vi "Main.vi"() -> ()   [LabVIEW 2020]
doc: "Ce VI modèle est conçu pour le modèle de conception Gestionnaire de messages dans une file d'attente.\n\nLa boucle de gestion d'événements génère des messages en fonction des actions sur l'interface utilisateur.\n\nLa boucle de gestion de messages traite les messages générés par la boucle de gestion d'événements ou par d'autres messages. Les messages sont des valeurs chaîne ; il est donc facile d'ajouter de nouveaux messages à la structure condition Conditions de messages de la boucle de gestion de messages Chaque cluster Message peut en outre fournir une valeur optionnelle pour Données de message, un variant qui peut être converti aux données requises pour un message spécifique."
uses:
  controls/UI Data.ctl
  support/Message Queue/All Message Queues.ctl
  support/Message Queue/Message Cluster.ctl
  controls/Display_Local.ctl
  support/Message Queue/Enqueue Message (Single).vi
  <vilib>/Utility/error.llb/Error Cluster From Error Code.vi
  <vilib>/ErrorRing/Error Ring.xnode
  support/Message Queue/Message Queue.lvlib
  support/User Event - Stop/User Event - Stop.lvlib
panel:
  in  "Cmd_Pad":T1
  in  "BTN_Error":bool
  in  "Btn_Arrêter":bool
  out "Ind_Display":T2
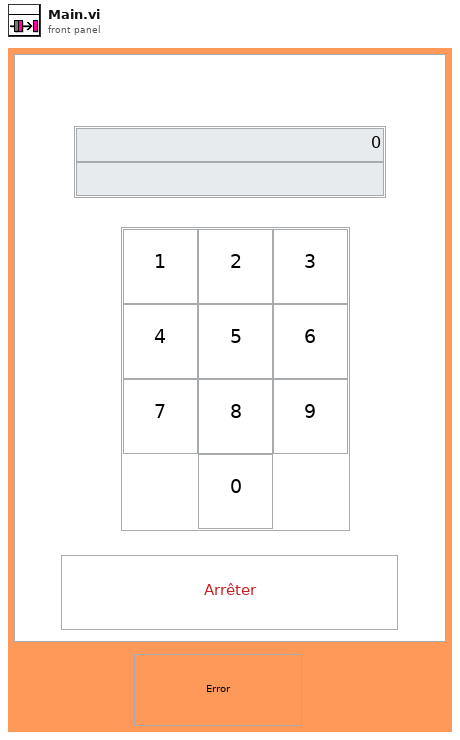
[diagram p1: front panel]
types:
  T1 = cluster{"Btn_1":bool, "Btn_2":bool, "Btn_3":bool, "Btn_4":bool, "Btn_5":bool, "Btn_6":bool, "Btn_7":bool, "Btn_8":bool, "Btn_9":bool, "Btn_10":bool}
  T2 = cluster{"Display_Numérique":dbl, "Display_Chaine":string}
  T3 = cluster{"état":bool, "code":i32, "source":string}
  T4 = typedef "Message Queue.lvlib/All Message Queues.ctl" = cluster{"IU":refnum<queue>, "CO":refnum<queue>}
  T5 = typedef "Display_Local.ctl" = cluster{"Display_Numérique":refnum<vi>, "Display_Chaine":refnum<vi>, "QMH":T4}
  T6 = typedef "UI Data.ctl" = cluster{"Char_Display":string, "Event_Stop ":refnum<user-event>, "QMH":T4}
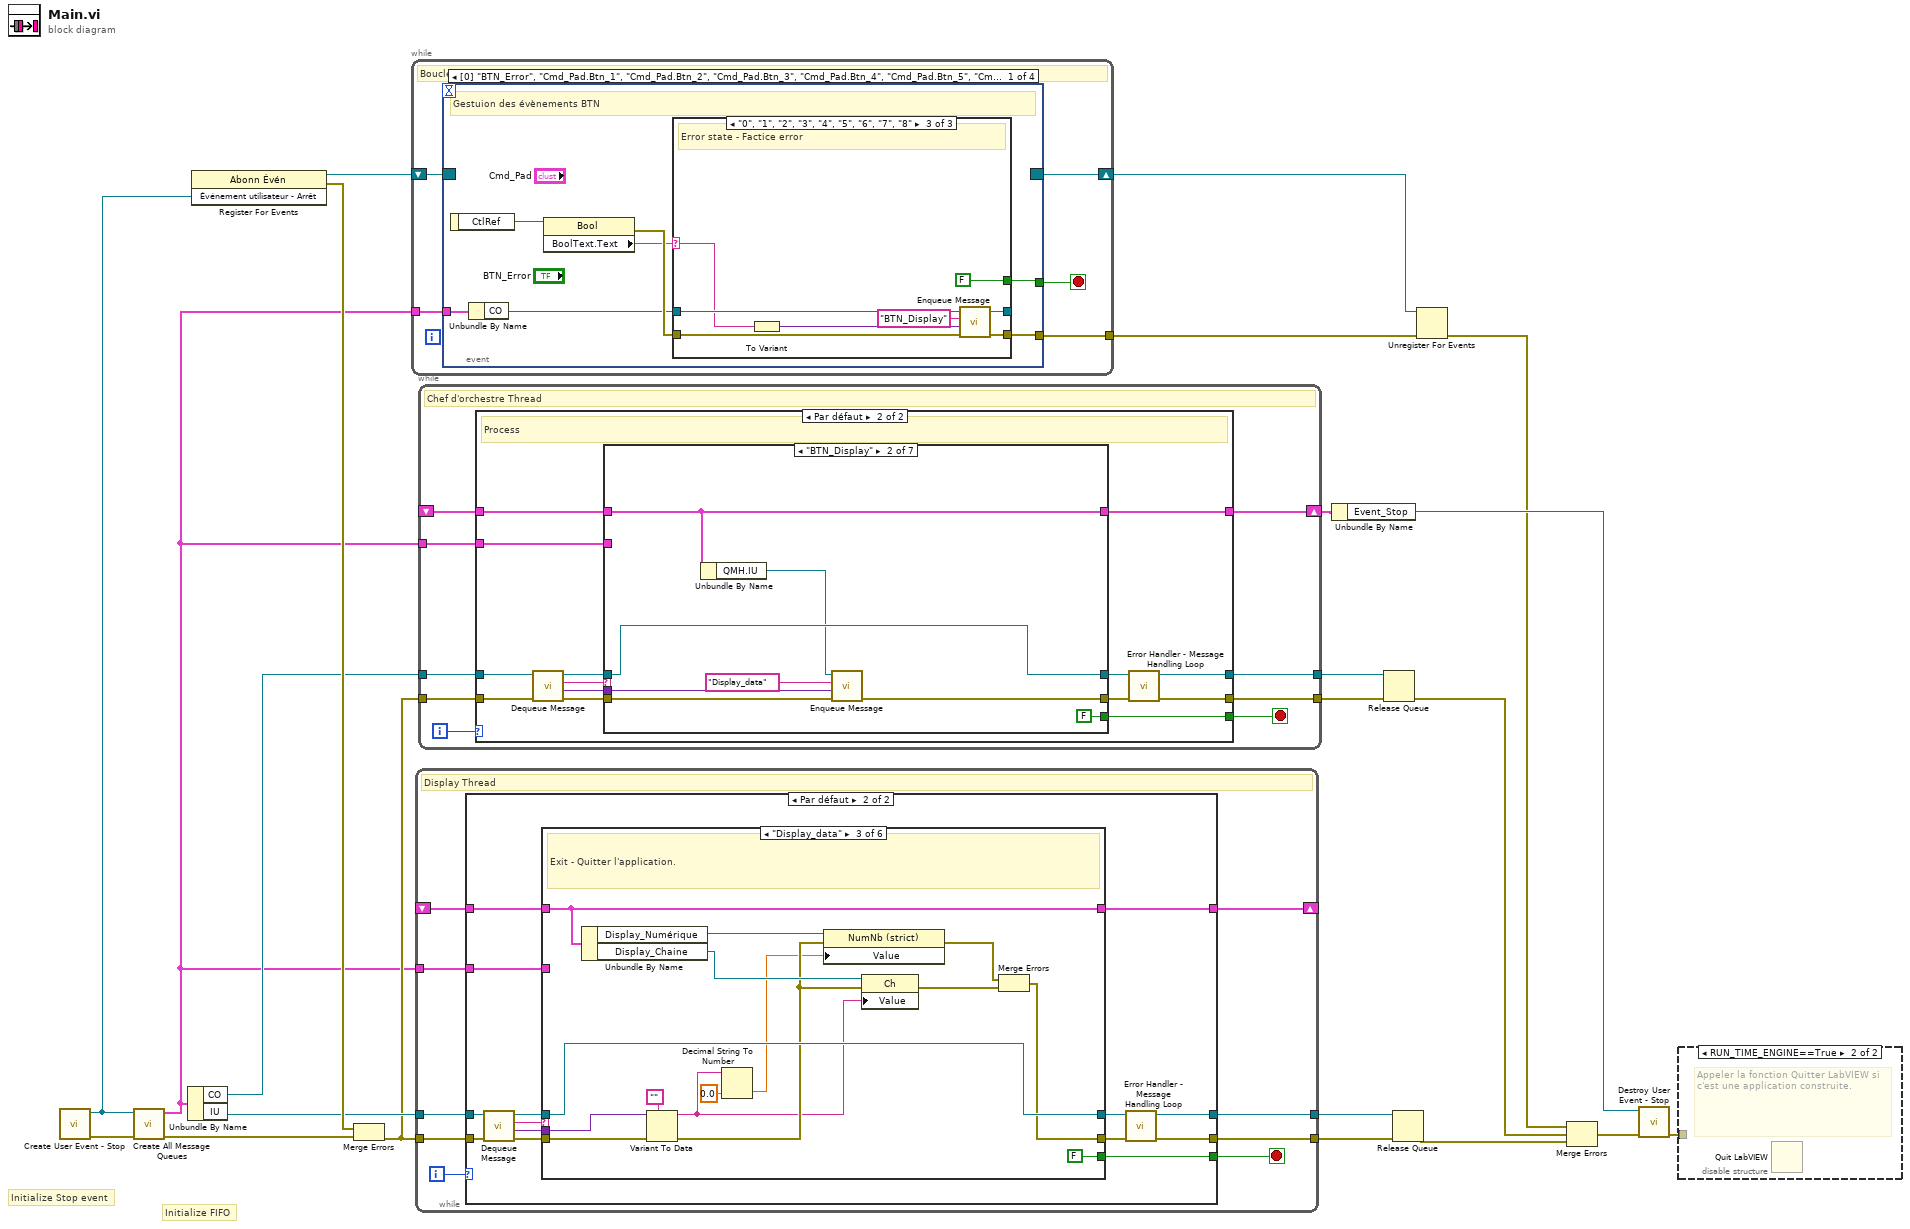
[diagram p0: block diagram]
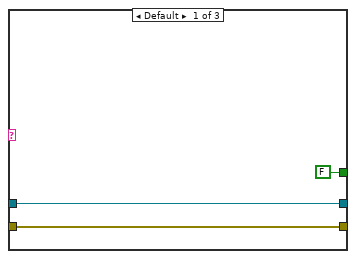
[diagram p2: hidden frame]
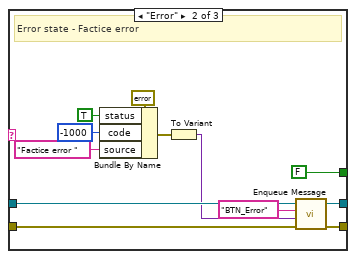
[diagram p3: hidden frame]
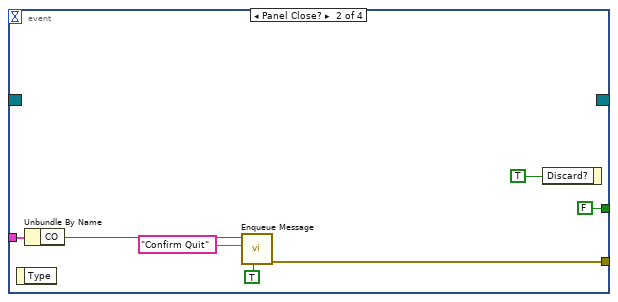
[diagram p4: hidden frame]
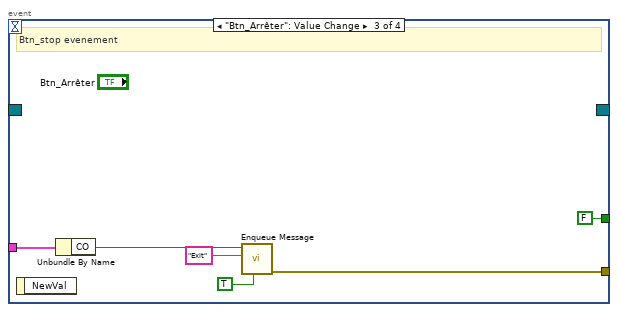
[diagram p5: hidden frame]
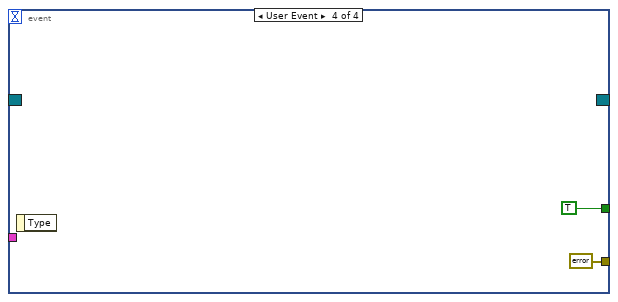
[diagram p6: hidden frame]
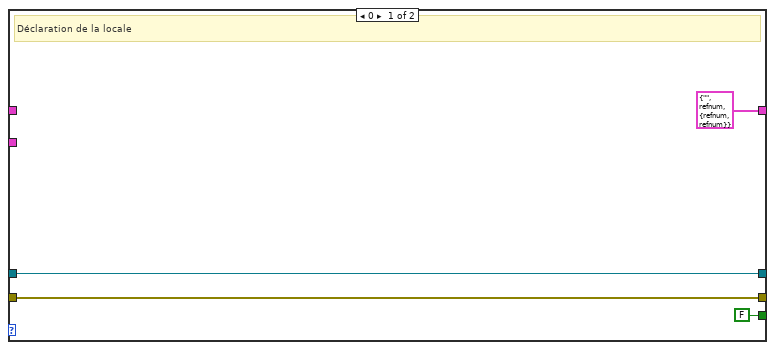
[diagram p7: hidden frame]
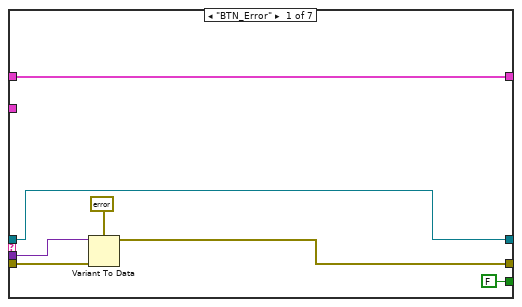
[diagram p8: hidden frame]
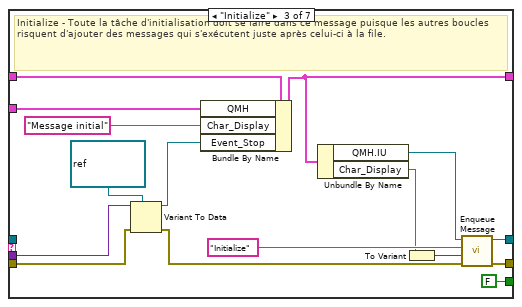
[diagram p9: hidden frame]
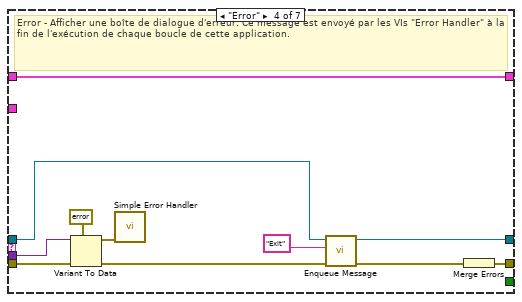
[diagram p10: hidden frame]
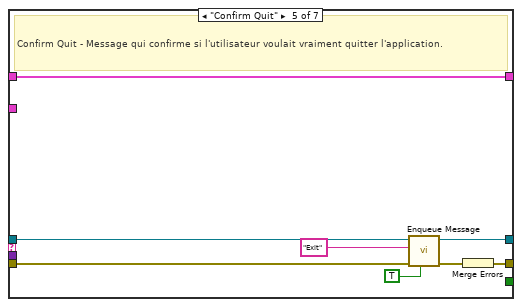
[diagram p11: hidden frame]
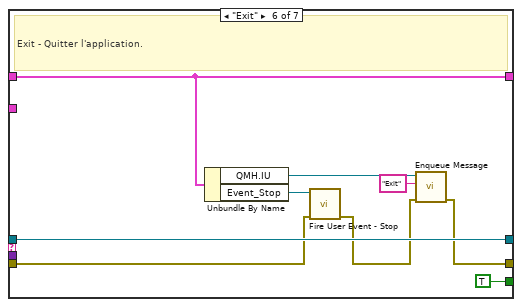
[diagram p12: hidden frame]
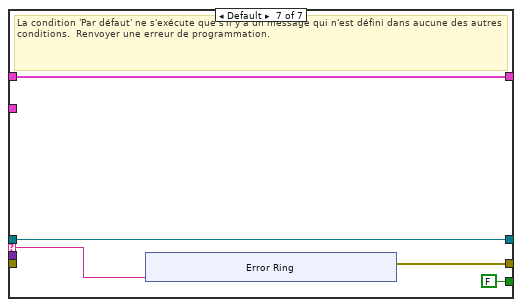
[diagram p13: hidden frame]
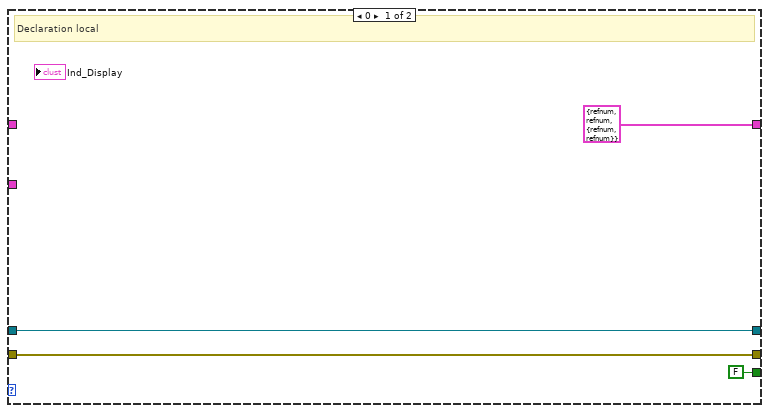
[diagram p14: hidden frame]
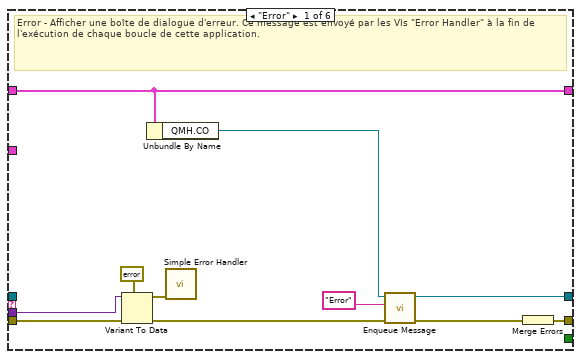
[diagram p15: hidden frame]
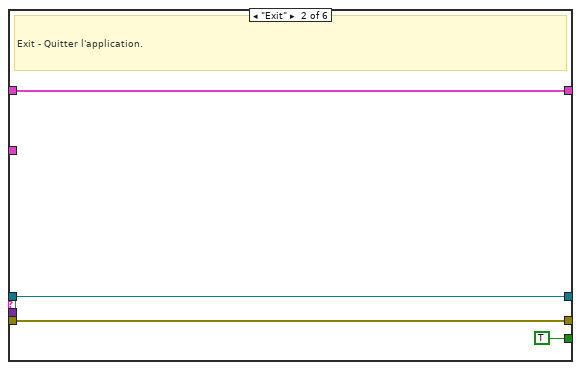
[diagram p16: hidden frame]
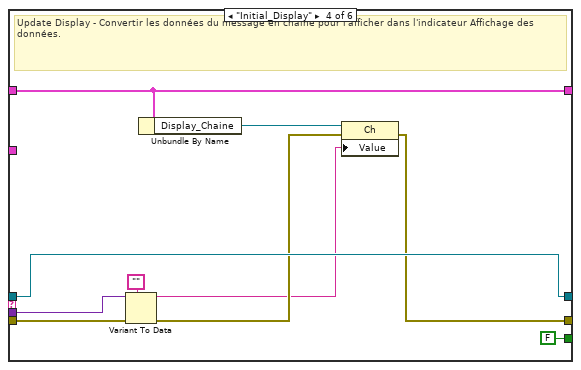
[diagram p17: hidden frame]
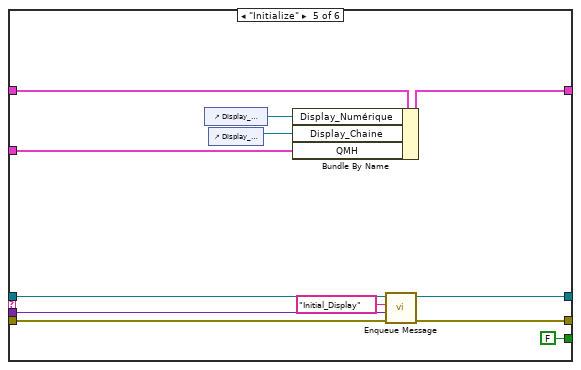
[diagram p18: hidden frame]
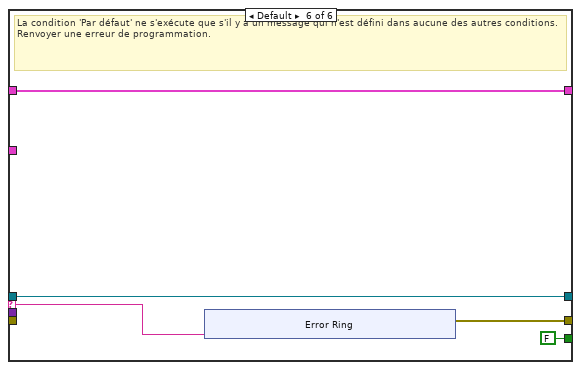
[diagram p19: hidden frame]
diagram:
  # "Initialize FIFO"
  # "Initialize Stop event"
  n1 = call "Create User Event - Stop.vi"() -> ("error out"=w21:T3, "Événement utilisateur - Arrêt"=w10:refnum<user-event>)  [unwired: 10 in]
  n2 = call "Create All Message Queues.vi"("error in (no error)"=w21, "Événement utilisateur - Arrêt"=w10) -> ("error out"=w22:T3, "Files d'attente de messages en sortie"=w5:T4)  [unwired: 8 in]
  n3 = Unbundle By Name(w5) -> ("CO"=w8:refnum<queue>, "IU"=w12:refnum<queue>)
  n4 = register-events(w10) -> (reference out=w16:refnum<event-registration>, error out=w15:errorcluster)  [unwired: 2 in]
  n5 = Merge Errors(w15, w22) -> (w9:errorcluster)
  n6 = while {
    tunnel: w5 -> [w27]
    shift-right: [w25] -> w19
    shift-left: w16 -> [w26]
    tunnel: [w23] -> w17
    stop <- w24 stop-if-true
    # "Boucle de gestion d'événements"
    n7 = event shown="[0] \"BTN_Error\", \"Cmd_Pad.Btn_1\", \"Cmd_Pad.Btn_2\", \"Cmd_Pad.Btn_3\", \"Cmd_Pad.Btn_4\", \"Cmd_Pad.Btn_5\", \"Cmd_Pad.Btn_6\", \"Cmd_Pad.Btn_7\", \"Cmd_Pad.Btn_8\", \"Cmd_Pad.Btn_9\", \"Cmd_Pad.Btn_10\": Valeur changée" {
      selector: w26 -> [_ _ _ _]
      dyn-events: [_ _ _ _] -> w25
      timeout: _ -> [_ _ _ _]
      tunnel: [w29 FALSE ("Discard?") FALSE ("Discard?") TRUE ("Discard?")] -> w24
      tunnel: w27 -> [w32 w63 w70 _]
      tunnel: [w31 w62 w69 T3 {"état"=FALSE, "code"=0, "source"=""} ("error out")] -> w23
      event "BTN_Error", "Cmd_Pad.Btn_1", "Cmd_Pad.Btn_2", "Cmd_Pad.Btn_3", "Cmd_Pad.Btn_4", "Cmd_Pad.Btn_5", "Cmd_Pad.Btn_6", "Cmd_Pad.Btn_7", "Cmd_Pad.Btn_8", "Cmd_Pad.Btn_9", "Cmd_Pad.Btn_10": Value Change {
        # "Gestuion des évènements BTN"
        n8 = event-data() -> ("CtlRef"=w34:refnum<vi>)  [unwired: 1 in]
        n9 = Unbundle By Name(w32) -> ("CO"=w28:refnum<queue>)
        n10 = property class="Bool"(reference=w34) -> (error out=w33:errorcluster, "BoolText.Text"=w30:string)  [unwired: 1 in, 1 out]
        n11 = case shown="\"0\", \"1\", \"2\", \"3\", \"4\", \"5\", \"6\", \"7\", \"8\"" w30 {
          selector: w30 -> [_ _ w52]
          tunnel: w33 -> [w36 w48 w57]
          tunnel: w28 -> [w37 w46 w55]
          tunnel: [w37 w45 w54] -> _
          tunnel: [w36 w47 w56] -> w31
          tunnel: [FALSE FALSE FALSE] -> w29
          frame Default {
          }
          frame "Error" {
            # "Error state - Factice error"
            n12 = Bundle By Name(cluster=errorcluster {"status"=FALSE, "code"=0, "source"=""} ("error out"), "status"=TRUE, "code"=-1000, "source"="Factice error ") -> (w40:errorcluster)
            n13 = To Variant(anything=w40) -> (Variant=w39:variant)
            n14 = call-poly "Enqueue Message.vi"("error in (no error)"=w48, "Données de message"=w39, "Message"="BTN_Error", "File d'attente de messages"=w46) -> ("error out"=w47:T3, "File d'attente de message dup."=w45:refnum<queue>)  [unwired: 6 in]
          }
          frame "0", "1", "2", "3", "4", "5", "6", "7", "8" {
            # "Error state - Factice error"
            n15 = To Variant(anything=w52) -> (Variant=w51:variant)
            n16 = call-poly "Enqueue Message.vi"("error in (no error)"=w57, "Données de message"=w51, "Message"="BTN_Display", "File d'attente de messages"=w55) -> ("error out"=w56:T3, "File d'attente de message dup."=w54:refnum<queue>)  [unwired: 6 in]
          }
        }
      }
      event Panel Close? {
        n17 = event-data() -> ()  [unwired: 1 in, 1 out]
        n18 = Unbundle By Name(w63) -> ("CO"=w58:refnum<queue>)
        n19 = call-poly "Enqueue Message.vi"("Message prioritaire ? (F)"=TRUE ("Priority Message? (F)"), "Message"="Confirm Quit", "File d'attente de messages"=w58) -> ("error out"=w62:T3)  [unwired: 7 in, 1 out]
        n20 = event-data ("Event Filter Node")("Discard?"=TRUE) -> ()  [unwired: 1 in, 1 out]
      }
      event "Btn_Arrêter": Value Change {
        # "Btn_stop evenement"
        n21 = event-data() -> ()  [unwired: 1 in, 1 out]
        n22 = Unbundle By Name(w70) -> ("CO"=w65:refnum<queue>)
        n23 = call-poly "Enqueue Message.vi"("Message prioritaire ? (F)"=TRUE ("Priority Message? (F)"), "Message"="Exit", "File d'attente de messages"=w65) -> ("error out"=w69:T3)  [unwired: 7 in, 1 out]
      }
      event User Event {
        n24 = event-data() -> ()  [unwired: 1 in, 1 out]
      }
    }
  }
  n25 = while {
    tunnel: w12 -> [w79]
    tunnel: w9 -> [w80]
    tunnel: [w78] -> w14
    tunnel: [w77] -> w11
    shift-right: [w75] -> _
    shift-left: _ -> [w74]
    tunnel: w5 -> [w73]
    i -> [w76]
    stop <- w81 stop-if-true
    # "Display Thread"
    n26 = case shown="Par défaut" w76 {
      tunnel: [FALSE w99] -> w81
      tunnel: w80 -> [w83 w98]
      tunnel: w79 -> [w84 w97]
      tunnel: [w83 w96] -> w78
      tunnel: [w84 w95] -> w77
      tunnel: [T5 {"Display_Numérique"=refnum, "Display_Chaine"=refnum, "QMH"={"IU"=refnum, "CO"=refnum}} ("Local_Display") w87] -> w75
      tunnel: w74 -> [_ w88]
      tunnel: w73 -> [_ w86]
      frame 0 {
        # "Declaration local"
      }
      frame Default {
        n27 = call "Dequeue Message.vi"("error in (no error)"=w98, "File d'attente de messages"=w97) -> ("error out"=w94:T3, "Données de message"=w92:variant, "Message"=w93:string, "File d'attente de message dup."=w91:refnum<queue>)  [unwired: 6 in]
        n28 = case "Conditions des messages" shown="\"Display_data\"" w93 {
          selector: w93 -> [_ _ _ _ _ w155]
          tunnel: w91 -> [_ w113 w125 w136 w143 w154]
          tunnel: w94 -> [w101 w112 w128 w139 w145 _]
          tunnel: [w110 w112 w118 w131 w146 w156] -> w90
          tunnel: [_ TRUE FALSE FALSE FALSE FALSE] -> w99
          tunnel: w92 -> [w102 _ w127 w138 w144 _]
          tunnel: [w107 w113 w125 w136 w142 w154] -> w89
          tunnel: w88 -> [w106 w111 w124 w134 w151 w152]
          tunnel: [w106 w111 w124 w134 w150 w152] -> w87
          tunnel: w86 -> [_ _ _ _ w140 _]
          frame "Error" {
            # "Error - Afficher une boîte de dialogue d'erreur. Ce message est envoyé par les VIs \"Error Handler\" à la fin de l'exécution de chaque boucle de cette application."
            n29 = Variant To Data(error in=w101, type=errorcluster {"status"=FALSE, "code"=0, "source"=""} ("error constant"), Variant=w102) -> (data=w104:errorcluster, error out=w100:errorcluster)
            n30 = Unbundle By Name(w106) -> ("QMH.CO"=w105:refnum<queue>)
            n31 = call <vilib>:"Simple Error Handler.vi"("error in (no error)"=w104) -> ()  [unwired: 4 in, 5 out]
            n32 = call-poly "Enqueue Message.vi"("error in (no error)"=w100, "Message"="Error", "File d'attente de messages"=w105) -> ("error out"=w108:T3, "File d'attente de message dup."=w107:refnum<queue>)  [unwired: 7 in]
            n33 = Merge Errors(w108) -> (w110:errorcluster)
          }
          frame "Exit" {
            # "Exit - Quitter l'application."
          }
          frame "Display_data" {
            # "Exit - Quitter l'application."
            n34 = Unbundle By Name(w124) -> ("Display_Numérique"=w123:refnum<vi>, "Display_Chaine"=w122:refnum<vi>)
            n35 = Variant To Data(error in=w128, type="", Variant=w127) -> (data=w117:string, error out=w121:errorcluster)
            n36 = Decimal String To Number(string=w117, default (0L)=0.0) -> (number=w116:dbl)  [unwired: 1 in, 1 out]
            n37 = property class="NumNb (strict)"(reference=w123, error in=w121, "Value"=w116) -> (error out=w120:errorcluster)  [unwired: 1 out]
            n38 = property class="Ch"(reference=w122, error in=w121, "Value"=w117) -> (error out=w119:errorcluster)  [unwired: 1 out]
            n39 = Merge Errors(w120, w119) -> (w118:errorcluster)
          }
          frame "Initial_Display" {
            # "Update Display - Convertir les données du message en chaîne pour l'afficher dans l'indicateur Affichage des données."
            n40 = Variant To Data(error in=w139, type="", Variant=w138) -> (data=w130:string, error out=w132:errorcluster)
            n41 = Unbundle By Name(w134) -> ("Display_Chaine"=w133:refnum<vi>)
            n42 = property class="Ch"(reference=w133, error in=w132, "Value"=w130) -> (error out=w131:errorcluster)  [unwired: 1 out]
          }
          frame "Initialize" {
            n43 = control-ref of="Display_Numérique"() -> (w149:refnum<vi>)
            n44 = control-ref of="Display_Chaine"() -> (w148:refnum<vi>)
            n45 = Bundle By Name(cluster=w151, "Display_Numérique"=w149, "Display_Chaine"=w148, "QMH"=w140) -> (w150:T5)
            n46 = call-poly "Enqueue Message.vi"("error in (no error)"=w145, "Données de message"=w144, "Message"="Initial_Display", "File d'attente de messages"=w143) -> ("error out"=w146:T3, "File d'attente de message dup."=w142:refnum<queue>)  [unwired: 6 in]
          }
          frame Default {
            # "La condition 'Par défaut' ne s'exécute que s'il y a un message qui n'est défini dans aucune des autres conditions.  Renvoyer une erreur de programmation."
            n47 = xnode ("Error Ring")("paramètre 0"=w155) -> ("sortie d'erreur"=w156:errorcluster)
          }
        }
        n48 = call "Error Handler - Message Handling Loop.vi"("error in (no error)"=w90, "File d'attente de messages"=w89) -> ("erreur en entrée dup."=w96:T3, "File d'attente de message dup."=w95:refnum<queue>)  [unwired: 8 in]
      }
    }
  }
  n49 = while {
    tunnel: w8 -> [w168]
    shift-right: [w171] -> w7
    shift-left: _ -> [w172]
    tunnel: w9 -> [w169]
    tunnel: [w167] -> w3
    tunnel: [w165] -> w4
    tunnel: w5 -> [w164]
    i -> [w166]
    stop <- w170 stop-if-true
    # "Chef d'orchestre Thread"
    n50 = case shown="Par défaut" w166 {
      tunnel: w172 -> [_ w190]
      tunnel: [T6 {"Char_Display"="", "Event_Stop "=refnum, "QMH"={"IU"=refnum, "CO"=refnum}} ("Data Cluster") w189] -> w171
      tunnel: [FALSE w188] -> w170
      tunnel: w169 -> [w175 w187]
      tunnel: w168 -> [w173 w183]
      tunnel: [w175 w181] -> w167
      tunnel: [w173 w178] -> w165
      tunnel: w164 -> [_ w177]
      frame 0 {
        # "Déclaration de la locale"
      }
      frame Default {
        # "Process"
        n51 = call "Dequeue Message.vi"("error in (no error)"=w187, "File d'attente de messages"=w183) -> ("error out"=w186:T3, "Données de message"=w184:variant, "Message"=w185:string, "File d'attente de message dup."=w182:refnum<queue>)  [unwired: 6 in]
        n52 = case "Conditions des messages" shown="\"BTN_Display\"" w185 {
          selector: w185 -> [_ _ _ _ _ _ w252]
          tunnel: w182 -> [w191 w204 _ w225 w236 w248 w251]
          tunnel: w186 -> [w196 w202 w215 w232 w240 w242 _]
          tunnel: [w192 w203 w221 w227 w238 w243 w253] -> w180
          tunnel: w190 -> [w197 w200 w220 w231 w239 w247 w254]
          tunnel: [w197 w200 w209 w231 w239 w247 w254] -> w189
          tunnel: [FALSE FALSE FALSE _ _ TRUE FALSE] -> w188
          tunnel: w184 -> [w193 w201 w211 w230 _ _ _]
          tunnel: [w191 w204 w217 w222 w233 w248 w251] -> w179
          tunnel: w177 -> [_ _ w210 _ _ _ _]
          frame "BTN_Error" {
            n53 = Variant To Data(error in=w196, type=errorcluster {"status"=FALSE, "code"=0, "source"=""} ("error out"), Variant=w193) -> (data=w192:errorcluster)  [unwired: 1 out]
          }
          frame "BTN_Display" {
            n54 = Unbundle By Name(w200) -> ("QMH.IU"=w199:refnum<queue>)
            n55 = call-poly "Enqueue Message.vi"("error in (no error)"=w202, "Données de message"=w201, "Message"="Display_data", "File d'attente de messages"=w199) -> ("error out"=w203:T3)  [unwired: 6 in, 1 out]
          }
          frame "Initialize" {
            # "Initialize - Toute la tâche d'initialisation doit se faire dans ce message puisque les autres boucles risquent d'ajouter des messages qui s'exécutent juste après celui-ci à la file."
            n56 = Variant To Data(error in=w215, type=refnum<user-event> refnum ("Événement utilisateur - Arrêt"), Variant=w211) -> (data=w213:refnum<user-event>, error out=w214:errorcluster)
            n57 = Bundle By Name(cluster=w220, "QMH"=w210, "Char_Display"="Message initial" ("Initial Message"), "Event_Stop"=w213) -> (w209:T6)
            n58 = Unbundle By Name(w209) -> ("QMH.IU"=w208:refnum<queue>, "Char_Display"=w207:string)
            n59 = To Variant(anything=w207) -> (Variant=w206:variant)
            n60 = call-poly "Enqueue Message.vi"("error in (no error)"=w214, "Données de message"=w206, "Message"="Initialize", "File d'attente de messages"=w208) -> ("error out"=w221:T3, "File d'attente de message dup."=w217:refnum<queue>)  [unwired: 6 in]
          }
          frame "Error" {
            # "Error - Afficher une boîte de dialogue d'erreur. Ce message est envoyé par les VIs \"Error Handler\" à la fin de l'exécution de chaque boucle de cette application."
            n61 = Variant To Data(error in=w232, type=errorcluster {"status"=FALSE, "code"=0, "source"=""} ("error constant"), Variant=w230) -> (data=w228:errorcluster, error out=w224:errorcluster)
            n62 = call <vilib>:"Simple Error Handler.vi"("error in (no error)"=w228) -> ()  [unwired: 4 in, 5 out]
            n63 = call-poly "Enqueue Message.vi"("error in (no error)"=w224, "Message"="Exit", "File d'attente de messages"=w225) -> ("error out"=w223:T3, "File d'attente de message dup."=w222:refnum<queue>)  [unwired: 7 in]
            n64 = Merge Errors(w223) -> (w227:errorcluster)
          }
          frame "Confirm Quit" {
            # "Confirm Quit - Message qui confirme si l'utilisateur voulait vraiment quitter l'application."
            n65 = call-poly "Enqueue Message.vi"("Message prioritaire ? (F)"=TRUE ("Priority Message? (F)"), "error in (no error)"=w240, "Message"="Exit", "File d'attente de messages"=w236) -> ("error out"=w237:T3, "File d'attente de message dup."=w233:refnum<queue>)  [unwired: 6 in]
            n66 = Merge Errors(w237) -> (w238:errorcluster)
          }
          frame "Exit" {
            # "Exit - Quitter l'application."
            n67 = Unbundle By Name(w247) -> ("QMH.IU"=w244:refnum<queue>, "Event_Stop"=w246:refnum<user-event>)
            n68 = call "Fire User Event - Stop.vi"("error in (no error)"=w242, "Événement utilisateur - Arrêt"=w246) -> ("error out"=w245:T3)  [unwired: 9 in]
            n69 = call-poly "Enqueue Message.vi"("error in (no error)"=w245, "Message"="Exit", "File d'attente de messages"=w244) -> ("error out"=w243:T3)  [unwired: 7 in, 1 out]
          }
          frame Default {
            # "La condition 'Par défaut' ne s'exécute que s'il y a un message qui n'est défini dans aucune des autres conditions.  Renvoyer une erreur de programmation."
            n70 = xnode ("Error Ring")("paramètre 0"=w252) -> ("sortie d'erreur"=w253:errorcluster)
          }
        }
        n71 = call "Error Handler - Message Handling Loop.vi"("error in (no error)"=w180, "File d'attente de messages"=w179) -> ("erreur en entrée dup."=w181:T3, "File d'attente de message dup."=w178:refnum<queue>)  [unwired: 8 in]
      }
    }
  }
  n72 = Unbundle By Name(w7) -> ("Event_Stop"=w6:refnum<user-event>)
  n73 = Release Queue(queue=w4, error in (no error)=w3) -> (error out=w1:errorcluster)  [unwired: 1 in, 2 out]
  n74 = Release Queue(queue=w11, error in (no error)=w14) -> (error out=w13:errorcluster)  [unwired: 1 in, 2 out]
  n75 = Unregister For Events(event registration refnum=w19, error in=w17) -> (error out=w2:errorcluster)
  n76 = Merge Errors(w2, w1, w13) -> (w20:errorcluster)
  n77 = call "Destroy User Event - Stop.vi"("error in (no error)"=w20, "Événement utilisateur - Arrêt"=w6) -> ("error out"=w18:T3)  [unwired: 9 in]
  n78 = disable-structure "Conditional Disable Structure" shown="RUN_TIME_ENGINE==True" {
    disable-tunnel: w18 -> [_ _]
    frame condition #0 (active) {
    }
    frame condition #1 {
      # "Appeler la fonction Quitter LabVIEW si c'est une application construite."
      n79 = Quit LabVIEW() -> ()  [unwired: 1 in]
    }
  }
